vi "create daemon config.vi"(8 "error in (no error)":errorcluster) -> (0 "error out":errorcluster)   [LabVIEW 2016, in "数据传输系统-04.lvlib" / "update.lvlib"]
uses:
  update.lvlib
  <vilib>/Utility/config.llb/Write Key (String).vi
  <vilib>/Utility/config.llb/NI_LVConfig.lvlib
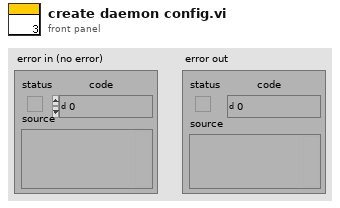
[diagram p1: front panel]
types:
  T1 = typedef "NI_LVConfig.lvlib/Config Data RefNum.ctl" = refnum<k1>
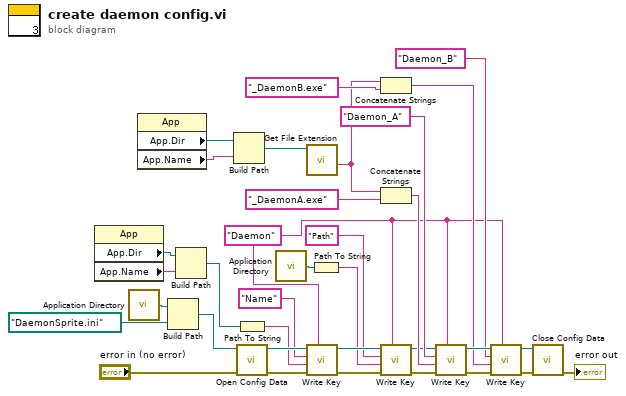
[diagram p0: block diagram]
diagram:
  w13 = "Daemon" ("section")
  n1 = property class="App"() -> ("App.Dir"=w8:path, "App.Name"=w7:string)  [unwired: 2 in, 2 out]
  n2 = call <vilib>:"Application Directory.vi"() -> ("Application Directory"=w34:path)
  n3 = property class="App"() -> ("App.Dir"=w3:path, "App.Name"=w2:string)  [unwired: 2 in, 2 out]
  n4 = Build Path(base path=w34, name or relative path=path "DaemonSprite.ini" ("Application Directory")) -> (appended path=w33:path)
  n5 = Build Path(base path=w8, name or relative path=w7) -> (appended path=w6:path)
  n6 = Build Path(base path=w3, name or relative path=w2) -> (appended path=w1:path)
  n7 = Path To String(path=w6) -> (string=w5:string)
  n8 = call <vilib>:"Open Config Data.vi"("error in (no error)"="error in (no error)", "configuration file path"=w33) -> ("error out"=w18:errorcluster, "refnum"=w17:T1)  [unwired: 7 in, 1 out]
  n9 = call <vilib>:"Application Directory.vi"() -> ("Application Directory"=w11:path)
  n10 = call <vilib>:"Get File Extension.vi"("file"=w1) -> ("filename without extension"=w26:string)  [unwired: 6 in, 4 out]
  n11 = call-poly <vilib>:"Write Key.vi"("section"=w13, "error in (no error)"=w18, "value"=w5, "key"="Name", "refnum"=w17) -> ("error out"=w15:errorcluster, "refnum out"=w14:T1)  [unwired: 4 in, 1 out]
  n12 = Path To String(path=w11) -> (string=w4:string)
  n13 = Concatenate Strings(w26, "_DaemonB.exe" ("名称或相对路径")) -> (w24:string)
  n14 = Concatenate Strings(w26, "_DaemonA.exe" ("名称或相对路径")) -> (w25:string)
  n15 = call-poly <vilib>:"Write Key.vi"("section"=w13, "error in (no error)"=w15, "value"=w4, "key"="Path", "refnum"=w14) -> ("error out"=w9:errorcluster, "refnum out"=w10:T1)  [unwired: 4 in, 1 out]
  n16 = call-poly <vilib>:"Write Key.vi"("section"=w13, "error in (no error)"=w9, "value"=w25, "key"="Daemon_A", "refnum"=w10) -> ("error out"=w31:errorcluster, "refnum out"=w32:T1)  [unwired: 4 in, 1 out]
  n17 = call-poly <vilib>:"Write Key.vi"("section"=w13, "error in (no error)"=w31, "value"=w24, "key"="Daemon_B", "refnum"=w32) -> ("error out"=w21:errorcluster, "refnum out"=w20:T1)  [unwired: 4 in, 1 out]
  n18 = call <vilib>:"Close Config Data.vi"("error in (no error)"=w21, "refnum"=w20) -> ("error out"=→"error out":errorcluster)  [unwired: 8 in, 1 out]
